vi "write to binary file.vi"() -> ()   [LabVIEW 2016]
uses:
  <vilib>/measure/NI_MABase.lvlib
panel:
  out "Waveform Graph":waveform(dbl)(graph)
  out "Data to file":dbl[](array[numeric])
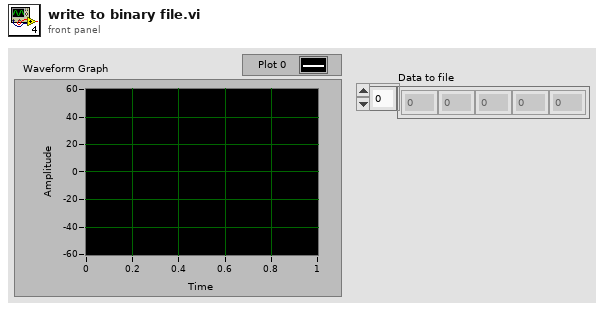
[diagram p1: front panel]
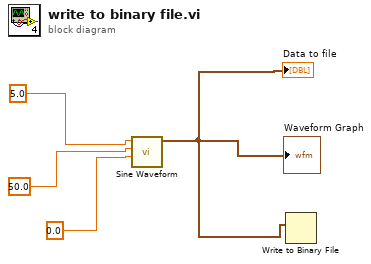
[diagram p0: block diagram]
diagram:
  n1 = call <vilib>:"Sine Waveform.vi"("phase"=0.0, "amplitude"=50.0, "frequency"=5.0) -> ("signal out"=w4:waveform(dbl))  [unwired: 7 in, 1 out]
  "Data to file" <- w4
  "Waveform Graph" <- w4
  n2 = Write to Binary File(data=w4) -> ()  [unwired: 5 in, 3 out]
